vi "testError.vi"() -> ()   [LabVIEW 2019, in "AssertionTest.lvlib" / "AssertStringContainsStringIgnoringCase.lvlib"]
uses:
  AssertStringContainsStringIgnoringCase.lvlib
  <vilib>/Utility/error.llb/Error Cluster From Error Code.vi
  <vilib>/ErrorRing/Error Ring.xnode
  Assertion/Assertion.lvlib
  36d383a9-d2e3-44af-afda-e2955e93e9be.vi
panel:
  out "error out":errorcluster
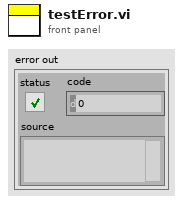
[diagram p1: front panel]
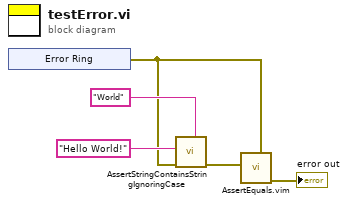
[diagram p0: block diagram]
diagram:
  n1 = xnode "Error Ring"() -> ("error out"=w2:errorcluster)
  n2 = call "AssertStringContainsStringIgnoringCase.vi"("Needle"="World", "error in (no error)"=w2, "Haystack"="Hello World!") -> ("error out"=w3:errorcluster)  [unwired: 8 in]
  n3 = call "AssertEquals.vim"("Expected"=w2, "Actual"=w3) -> ("error out"=→"error out":errorcluster)  [unwired: 9 in]
